vi "Hormiga_pinMode.vi"(8 "error in (no error)":errorcluster, 9 "GPIO Mode":enum16{"OUTPUT", "INPUT"}(ring), 10 "Terminal":u8=13, 11 "VISA Refnum in":refnum<visa-resource-name>) -> (0 "error out":errorcluster, 2 "Returned Value":u8, 3 "VISA Refnum out":refnum<visa-resource-name>)   [LabVIEW 2016]
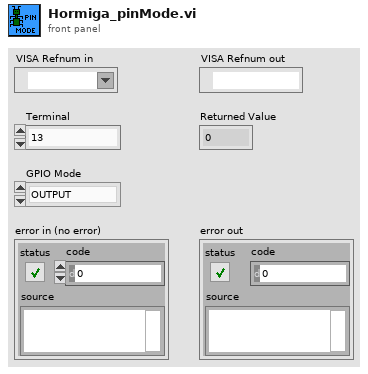
[diagram p1: front panel]
types:
  T1 = enum16{"pinMode", "digitalWrite", "digitalRead", "analogRead", "analogWrite"}
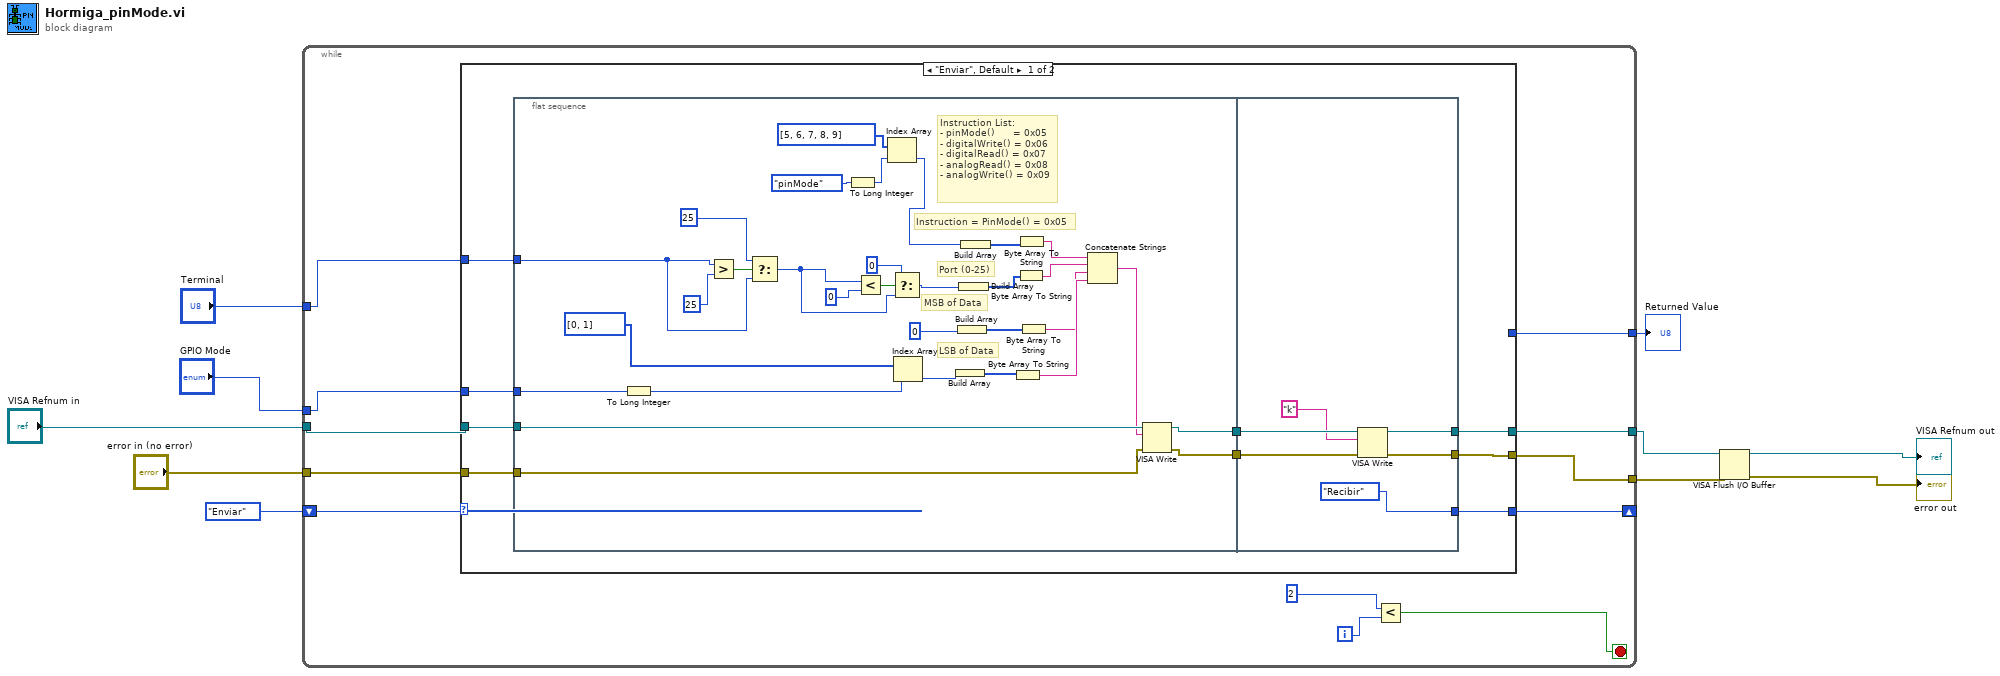
[diagram p0: block diagram]
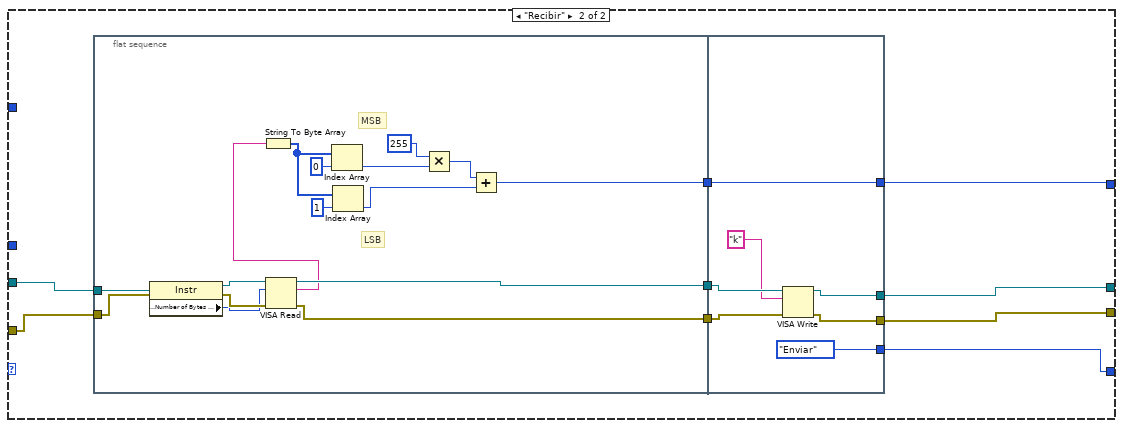
[diagram p2: hidden frame]
diagram:
  n1 = while {
    shift-right: [w17] -> _
    shift-left: enum16{"Enviar", "Recibir"}."Enviar" -> [w22]
    tunnel: "error in (no error)" -> [w21]
    tunnel: "VISA Refnum in" -> [w20]
    tunnel: [w19] -> w4
    tunnel: [w18] -> w2
    tunnel: "Terminal" -> [w13]
    tunnel: "GPIO Mode" -> [w12]
    tunnel: [w11] -> w10
    i -> [w15]
    stop <- w16 stop-if-true
    n2 = case shown="\"Enviar\", Default" w22 {
      tunnel: w21 -> [w31 w77]
      tunnel: w20 -> [w30 w76]
      tunnel: [w27 w73] -> w19
      tunnel: [w26 w72] -> w18
      tunnel: [w25 w71] -> w17
      tunnel: w13 -> [w24 _]
      tunnel: w12 -> [w23 _]
      tunnel: [_ w69] -> w11
      frame "Enviar", Default {
        n3 = flat-sequence {
          tunnel: w31 -> [w62]
          tunnel: w30 -> [w61]
          tunnel: [w60] -> w29
          tunnel: [w59] -> w28
          tunnel: w24 -> [w34]
          tunnel: w23 -> [w33]
          tunnel: w29 -> [w68]
          tunnel: w28 -> [w67]
          tunnel: [w65] -> w27
          tunnel: [w64] -> w26
          tunnel: [enum16{"Enviar", "Recibir"}."Recibir"] -> w25
          frame #0 {
            # "Instruction List:\n- pinMode()      = 0x05\n- digitalWrite() = 0x06\n- digitalRead() = 0x07\n- analogRead() = 0x08\n- analogWrite() = 0x09"
            # "LSB of Data"
            # "MSB of Data"
            # "Port (0-25)"
            # "Instruction = PinMode() = 0x05"
            n4 = To Long Integer(number=w33) -> (32bit integer=w36:i32)
            n5 = Greater?(x=w34, y=u8 25) -> (0:w44:bool)
            n6 = Select(t=u8 25, s=w44, f=w34) -> (s? t:f=w39:u8)
            n7 = To Long Integer(number=T1."pinMode") -> (32bit integer=w47:i32)
            n8 = Less?(x=w39, y=u8 0) -> (x < y?=w41:bool)
            n9 = Index Array(array=u8[] [5, 6, 7, 8, 9], index=w47) -> (element=w46:u8)
            n10 = Select(t=u8 0, s=w41, f=w39) -> (s? t:f=w38:u8)
            n11 = Index Array(array=u8[] [0, 1], index=w36) -> (element=w35:u8)
            n12 = Build Array(w35) -> (w54:u8[])
            n13 = Build Array(u8 0) -> (w55:u8[])
            n14 = Build Array(w38) -> (w56:u8[])
            n15 = Build Array(w46) -> (w57:u8[])
            n16 = Byte Array To String(unsigned byte array=w54) -> (string=w53:string)
            n17 = Byte Array To String(unsigned byte array=w56) -> (string=w51:string)
            n18 = Byte Array To String(unsigned byte array=w57) -> (string=w50:string)
            n19 = Byte Array To String(unsigned byte array=w55) -> (string=w52:string)
            n20 = Concatenate Strings(w50, w51, w52, w53) -> (w32:string)
            n21 = VISA Write(VISA resource name=w61, write buffer=w32, error in (no error)=w62) -> (VISA resource name out=w59:refnum<visa-resource-name>, error out=w60:errorcluster)  [unwired: 1 out]
          }
          frame #1 {
            n22 = VISA Write(VISA resource name=w67, write buffer="k", error in (no error)=w68) -> (VISA resource name out=w64:refnum<visa-resource-name>, error out=w65:errorcluster)  [unwired: 1 out]
          }
        }
      }
      frame "Recibir" {
        n23 = flat-sequence {
          tunnel: w77 -> [w93]
          tunnel: w76 -> [w92]
          tunnel: [w88] -> w75
          tunnel: [w87] -> w74
          tunnel: [w78] -> w70
          tunnel: w75 -> [w100]
          tunnel: w74 -> [w99]
          tunnel: [w97] -> w73
          tunnel: [w96] -> w72
          tunnel: [enum16{"Enviar", "Recibir"}."Enviar"] -> w71
          tunnel: w70 -> [w94]
          tunnel: [w94] -> w69
          frame #0 {
            # "MSB"
            # "LSB"
            n24 = property class="Instr"(reference=w92, error in=w93) -> (reference out=w90:refnum<visa-resource-name>, error out=w91:errorcluster, "Serial Settings:Number of Bytes at Serial Port"=w89:u32)
            n25 = VISA Read(VISA resource name=w90, byte count=w89, error in (no error)=w91) -> (VISA resource name out=w87:refnum<visa-resource-name>, read buffer=w86:string, error out=w88:errorcluster)  [unwired: 1 out]
            n26 = String To Byte Array(string=w86) -> (unsigned byte array=w85:u8[])
            n27 = Index Array(array=w85, index=0) -> (element=w82:u8)
            n28 = Index Array(array=w85, index=1) -> (element=w79:u8)
            n29 = Multiply(x=u8 255, y=w82) -> (x*y=w81:u8)
            n30 = Add(x=w81, y=w79) -> (x+y=w78:u8)
          }
          frame #1 {
            n31 = VISA Write(VISA resource name=w99, write buffer="k", error in (no error)=w100) -> (VISA resource name out=w96:refnum<visa-resource-name>, error out=w97:errorcluster)  [unwired: 1 out]
          }
        }
      }
    }
    n32 = Less?(x=2, y=w15) -> (x < y?=w16:bool)
  }
  "Returned Value" <- w10
  n33 = VISA Flush I/O Buffer(VISA resource name=w2, error in (no error)=w4) -> (VISA resource name out=→"VISA Refnum out":refnum<visa-resource-name>, error out=→"error out":errorcluster)  [unwired: 1 in]
